vi "Set PDOs COB IDs.vi"(6 "Node ID":u32, 7 "timeout (1s)":dbl=1.0 min=0.0, 8 "error in (no error)":errorcluster, 11 "SDO object in":refnum<k20>) -> (0 "error out":errorcluster, 3 "SDO object out":refnum<k20>)   [LabVIEW 2016]
uses:
  <vilib>/CANopenLib/CANOPEN.llb/CANopen SDO Write [U32].vi
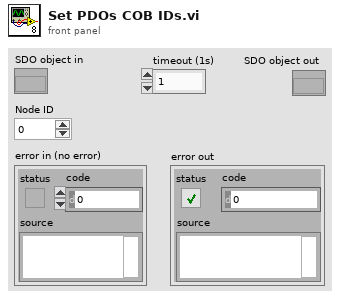
[diagram p1: front panel]
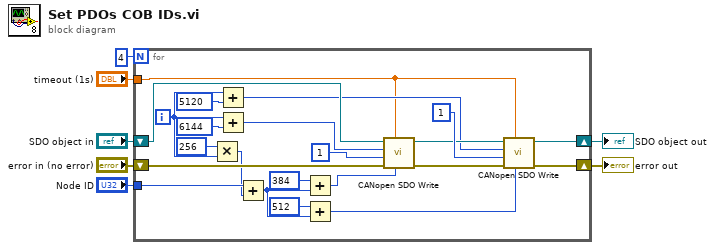
[diagram p0: block diagram]
diagram:
  n1 = for {
    N: 4 -> [_]
    tunnel: "Node ID" -> [w16]
    shift-right: [w28] -> w5
    shift-left: "error in (no error)" -> [w29]
    shift-right: [w18] -> w3
    shift-left: "SDO object in" -> [w27]
    tunnel: "timeout (1s)" -> [w8]
    i -> [w9]
    n2 = Multiply(x=u32 256, y=w9) -> (x*y=w15:u32)
    n3 = Add(x=w9, y=u16 5120 ("object index")) -> (x+y=w10:i32)
    n4 = Add(x=w9, y=u16 6144 ("object index")) -> (x+y=w12:i32)
    n5 = Add(x=w16, y=w15) -> (x+y=w14:u32)
    n6 = Add(x=u32 384, y=w14) -> (x+y=w22:u32)
    n7 = Add(x=u32 512, y=w14) -> (x+y=w21:u32)
    n8 = call-poly <vilib>:"CANopen SDO Write.vi"("U32 data"=w22, "timeout (1s)"=w8, "error in (no error)"=w29, "object sub-index (0)"=u8 1, "object index"=w12, "SDO object in"=w27) -> ("error out"=w20:errorcluster, "SDO object out"=w19:refnum<k20>)  [unwired: 3 in, 1 out]
    n9 = call-poly <vilib>:"CANopen SDO Write.vi"("U32 data"=w21, "timeout (1s)"=w8, "error in (no error)"=w20, "object sub-index (0)"=u8 1, "object index"=w10, "SDO object in"=w19) -> ("error out"=w28:errorcluster, "SDO object out"=w18:refnum<k20>)  [unwired: 3 in, 1 out]
  }
  "error out" <- w5
  "SDO object out" <- w3
